vi "spectral_inspect.vi"(8 "error in (no error)":errorcluster, 11 "waveform":waveform(dbl)) -> (0 "Csapásszám [stroke/min]":dbl, 1 "freq":dbl, 2 "amplitude":dbl, 3 "PSD":cluster{"f0":dbl, "df":dbl, "magnitude":dbl[]}(graph), 4 "error out":errorcluster)   [LabVIEW 2020]
uses:
  <vilib>/express/express analysis/Spectral/Block/exnSpectralBlock spectral measurements PSD poly.vi
  <vilib>/express/express analysis/Spectral/Block/exnSpectralBlock spectral measurements PSD WFM.vi
  <vilib>/express/express analysis/Spectral/XNode/ExpressSpectralMeasurementsBlockNode.xnode
panel:
  out "Waveform Chart":waveform(dbl)(graph)
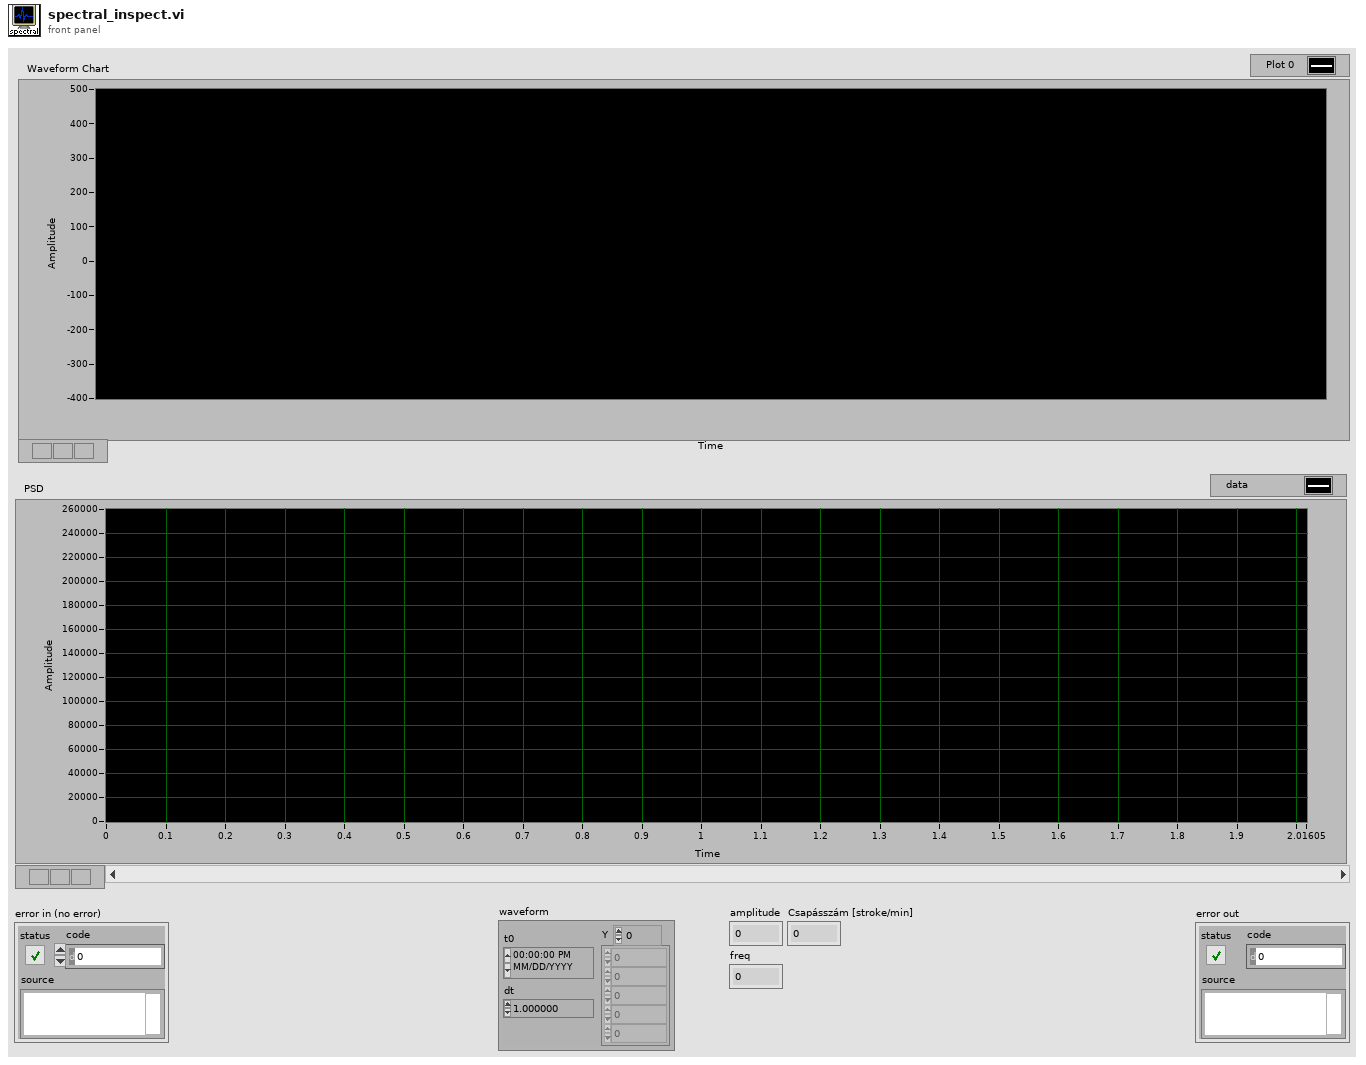
[diagram p1: front panel]
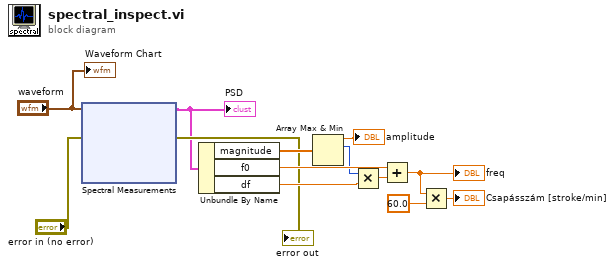
[diagram p0: block diagram]
diagram:
  n1 = xnode "Spectral Measurements"("Signals"="waveform", "error in (no error)"="error in (no error)") -> ("PSD"=w1:cluster{"f0":dbl, "df":dbl, "magnitude":dbl[]}, "error out"=→"error out":errorcluster)
  "PSD" <- w1
  n2 = Unbundle By Name(w1) -> ("magnitude"=w13:dbl[], "f0"=w11:dbl, "df"=w9:dbl)
  n3 = Array Max & Min(array=w13) -> (max value=→"amplitude":dbl, max index (indices)=w10:i32)  [unwired: 2 out]
  n4 = Multiply(x=w10, y=w9) -> (x*y=w8:dbl)
  n5 = Add(x=w11, y=w8) -> (x+y=w5:dbl)
  "freq" <- w5
  n6 = Multiply(x=w5, y=60.0) -> (x*y=→"Csapásszám [stroke/min]":dbl)
  "Waveform Chart" <- "waveform"
